vi "protection-mainSD.vi"(1 "error in (no error)":errorcluster, 2 "Cluster":T1) -> (0 "error out":errorcluster)   [LabVIEW 2015]
uses:
  controls/protection-cluster.ctl
  controls/Daqmxtasks.ctl
  globalVarSD.vi
panel:
  in  "Path sound of alarm":path=path "S:/TRANCON/sounds/swgzq-rkyg3.wav"
  in  "current Alarm break, uA":dbl=100.0 format="%#_13g"
  in  "current Alarm, uA":dbl=1000.0 format="%#_13g"
  out "Alarm current":dbl
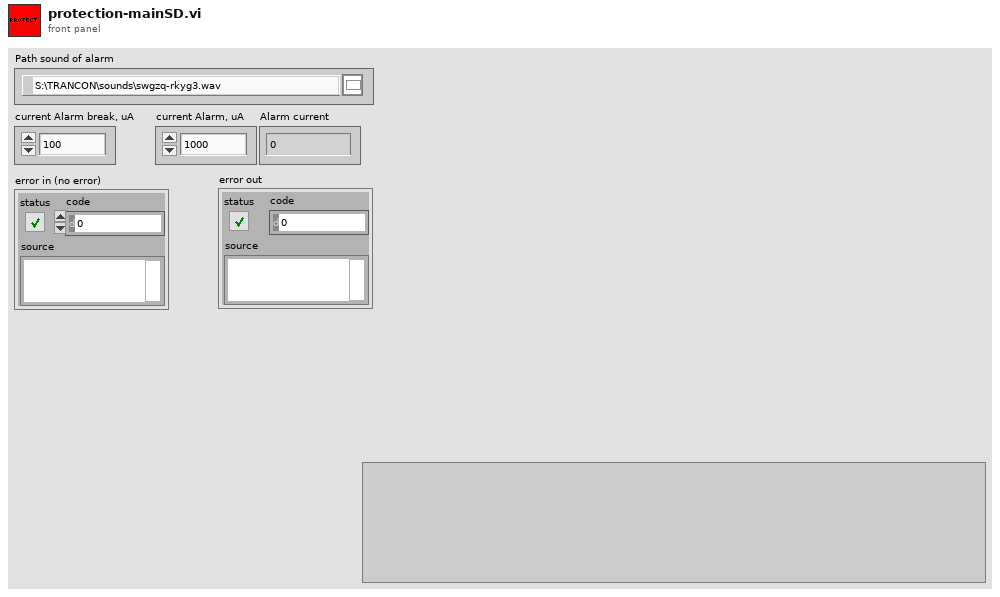
[diagram p1: front panel]
types:
  T1 = typedef "protection-cluster.ctl" = cluster{"Stop event":refnum<event-registration>, "Block accelerator":refnum<vi>, "Accelerator protected":refnum<vi>, "Relay key":refnum<vi>, "cluster of DAQ tasks":T2, "ALARM":refnum<vi>}
  T2 = typedef "Daqmxtasks.ctl" = cluster{"Heater alaram task":refnum<k21>, "Laser shutter task":refnum<k21>, "Motor task":refnum<k21>, "Accelerator shutter task":refnum<k21>, "Relay key task":refnum<k21>, "Faraday cup task":refnum<k21>}
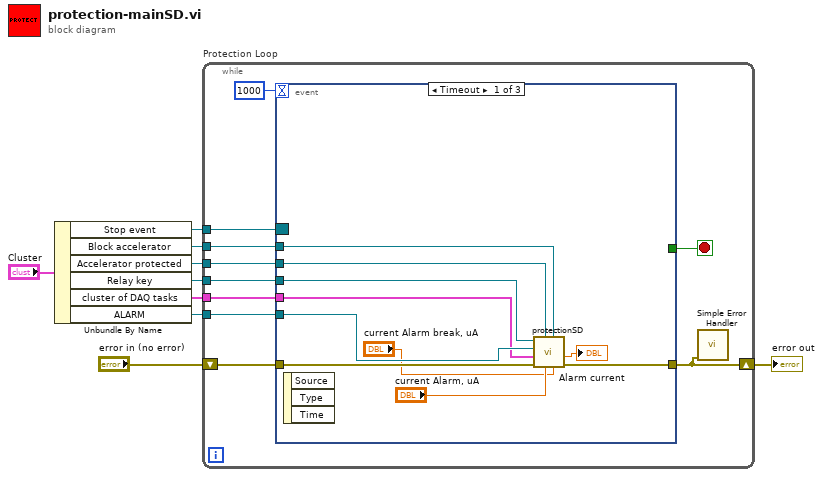
[diagram p0: block diagram]
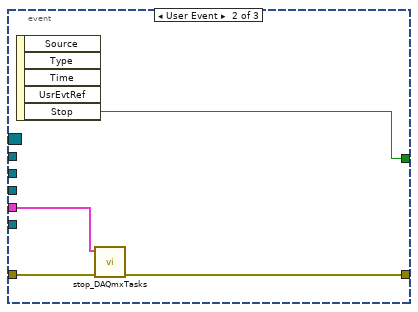
[diagram p2: hidden frame]
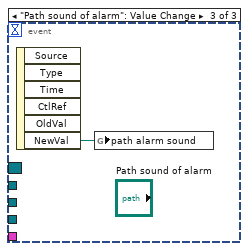
[diagram p3: hidden frame]
diagram:
  n1 = Unbundle By Name("Cluster") -> ("Stop event"=w6:refnum<event-registration>, "Block accelerator"=w5:refnum<vi>, "Accelerator protected"=w4:refnum<vi>, "Relay key"=w3:refnum<vi>, "cluster of DAQ tasks"=w2:T2, "ALARM"=w1:refnum<vi>)
  n2 = while "Protection Loop" {
    shift-right: [w16] -> w8
    shift-left: "error in (no error)" -> [w17]
    tunnel: w6 -> [w15]
    tunnel: w2 -> [w14]
    tunnel: w5 -> [w11]
    tunnel: w3 -> [w13]
    tunnel: w1 -> [w12]
    tunnel: w4 -> [w10]
    stop <- w19 stop-if-true
    n3 = event shown="[0] Timeout" {
      selector: w15 -> [_ _ _]
      dyn-events: _ -> [_ _ _]
      timeout: 1000 -> [_ _ _]
      tunnel: [_ w33 _] -> w19
      tunnel: [w28 w32 _] -> w16
      tunnel: w17 -> [w29 w31 _]
      tunnel: w14 -> [w22 w30 _]
      tunnel: w13 -> [w27 _ _]
      tunnel: w12 -> [w26 _ _]
      tunnel: w11 -> [w21 _ _]
      tunnel: w10 -> [w20 _ _]
      event Timeout {
        n4 = event-data() -> ()  [unwired: 1 in, 3 out]
        n5 = call "protectionSD.vi"("current Alarm break, uA"="current Alarm break, uA", "Block accelerator"=w21, "current Alarm, uA"="current Alarm, uA", "Accelerator protected"=w20, "error in (no error)"=w29, "cluster of DAQ tasks"=w22, "Alarm Refnum"=w26, "Relay key refnum"=w27) -> ("error out"=w28:errorcluster, "Alarm current"=→"Alarm current":dbl)  [unwired: 2 in]
      }
      event User Event {
        n6 = event-data() -> ("Stop"=w33:bool)  [unwired: 1 in, 4 out]
        n7 = call "stop_DAQmxTasks.vi"("error in (no error)"=w31, "cluster of DAQ tasks"=w30) -> ("error out"=w32:errorcluster)  [unwired: 9 in]
      }
      event "Path sound of alarm": Value Change {
        n8 = event-data() -> ("NewVal"=w34:path)  [unwired: 1 in, 5 out]
        n9 = global write "globalVarSD.vi" "path alarm sound"(w34) -> ()
      }
    }
    n10 = call <vilib>:"Simple Error Handler.vi"("error in (no error)"=w16) -> ()  [unwired: 4 in, 5 out]
  }
  "error out" <- w8
